vi "apolin.vi"() -> ()   [LabVIEW 2014]
uses:
  <vilib>/Platform/TimedLoop/XDataNode/timing_clust.ctl
  <vilib>/Platform/TimedLoop/XDataNode/nitl_modes.ctl
  <vilib>/Platform/TimedLoop/XDataNode/wakeup.ctl
  <vilib>/myRIO/Instrument Drivers/Onboard IO/AO/typedefs/AO Reference.ctl
  <vilib>/myRIO/Common/Instrument Driver Framework/Utilities/typedefs/myRIO Generic Hardware Reference.ctl
  <vilib>/myRIO/Common/Instrument Driver Framework/Utilities/typedefs/Hardware Version Enum.ctl
  <vilib>/myRIO/Common/Instrument Driver Framework/Utilities/typedefs/myRIO v1.0 Reference.ctl
  <vilib>/myRIO/Common/Instrument Driver Framework/Utilities/typedefs/Generic FPGA Reference.ctl
  <vilib>/myRIO/Common/Instrument Driver Framework/myRIO v1.0/AO/typedefs/AO Channels List.ctl
  <vilib>/myRIO/Common/Instrument Driver Framework/myRIO v1.0/AO/typedefs/AO Channels Enum.ctl
  <vilib>/myRIO/Common/Instrument Driver Framework/Utilities/typedefs/Analog Scaling Constants List.ctl
  <vilib>/myRIO/Common/Instrument Driver Framework/Utilities/typedefs/Analog Scaling Constants.ctl
  <vilib>/userdefined/High Color/nirio_resource_hc.ctl
  <vilib>/myRIO/Common/Instrument Driver Framework/myRIO v1.0/AO/vis/myRIO v1.1 Open AO.vi
  <vilib>/myRIO/Common/Instrument Driver Framework/Utilities/vis/Validate Channels.vi
  <vilib>/myRIO/Common/Instrument Driver Framework/myRIO v1.0/AO/vis/myRIO v1.0 Reserve AO.vi
  <vilib>/myRIO/Common/Instrument Driver Framework/myRIO v1.0/AO/vis/myRIO v1.0 Close AO.vi
  <vilib>/myRIO/Common/Instrument Driver Framework/myRIO v1.0/AO/vis/myRIO v1.0 Build MUX Configuration AO.vi
  <vilib>/myRIO/Common/Instrument Driver Framework/myRIO v1.0/Resource Manager/vis/myRIO v1.0 Reserve Channel List.vi
  <vilib>/myRIO/Common/Instrument Driver Framework/myRIO v1.0/AO/vis/myRIO v1.0 Unreserve AO.vi
  <vilib>/myRIO/Common/Instrument Driver Framework/myRIO v1.0/Resource Manager/vis/myRIO v1.0 Reserve Channel.vi
  <vilib>/myRIO/Common/Instrument Driver Framework/myRIO v1.0/Resource Manager/vis/myRIO v1.0 Unreserve Channel.vi
  <vilib>/myRIO/Common/Instrument Driver Framework/myRIO v1.0/Resource Manager/vis/myRIO v1.0 Unreserve Channel List.vi
  <vilib>/myRIO/Common/Instrument Driver Framework/myRIO v1.0/Resource Manager/vis/myRIO v1.0 Build Mutex Name.vi
  <vilib>/Utility/VariantDataType/GetNumericInfo.vi
  <vilib>/Utility/error.llb/Error Cluster From Error Code.vi
  <vilib>/myRIO/Common/Instrument Driver Framework/myRIO v1.0/myRIO v1.1 Open.vi
  <vilib>/myRIO/Common/Instrument Driver Framework/myRIO v1.0/AO/vis/myRIO v1.0 Get Scaling Constants AO.vi
  <vilib>/myRIO/Common/Instrument Driver Framework/Utilities/vis/IO Manager.vi
  <vilib>/myRIO/Common/Instrument Driver Framework/Utilities/vis/Configuration Manager.vi
  <vilib>/myRIO/Common/Instrument Driver Framework/myRIO v1.0/myRIO v1.0 Close.vi
  <vilib>/myRIO/Common/Instrument Driver Framework/myRIO v1.0/AO/vis/myRIO v1.0 Write AO.vi
  <vilib>/myRIO/Instrument Drivers/Onboard IO/AO/vis/myRIO AO Open.xnode
  <vilib>/platform/TimedLoop/XDataNode/XDataNode.xnode
  <vilib>/myRIO/Common/Instrument Driver Framework/myRIO v1.0/AI/typedefs/AI Channels Enum.ctl
  <vilib>/myRIO/Common/Instrument Driver Framework/myRIO v1.0/AI/typedefs/AI Channels List.ctl
  <vilib>/myRIO/Instrument Drivers/Onboard IO/AI/typedefs/AI Reference.ctl
  <vilib>/myRIO/Instrument Drivers/Onboard IO/AI/AI.lvlib
  <vilib>/myRIO/Common/Instrument Driver Framework/myRIO v1.0/AI/vis/myRIO v1.1 Open AI.vi
  <vilib>/myRIO/Instrument Drivers/Onboard IO/AI/vis/myRIO AI Open.xnode
  <vilib>/Platform/TimedLoop/XDataNode/XDNodeRunTimeDep.lvlib
  <vilib>/myRIO/Instrument Drivers/Onboard IO/AO/AO.lvlib
  <vilib>/measure/NI_MABase.lvlib
panel:
  out "x/y":dbl
  in  "Start \nPlayback":bool
  out "Recording 3":dbl[](graph)
  out "Array 3":dbl[][](array[numeric])
  in  "sampling info":cluster{"Fs":dbl, "#s":dbl}={"Fs"=40000.0, "#s"=40000.0} {"Fs" format="%.2p"}
  out "error out":errorcluster
  out "dt":dbl
  in  "tones":T1(array[cluster])=[{"frequency"=10.0, "amplitude"=1.0, "phase"=0.0}, {"frequency"=20.0, "amplitude"=0.1, "phase"=0.0}] {"phase" format="%.2p"; "amplitude" format="%0.2p"; "frequency" format="%0.2p"}
  in  "Stop \nPlaying":bool
  out "Array":dbl[](array[numeric])
  out "Recording 2":dbl(graph)
  in  "Stop \nRecording 2":bool
  out "Array 2":dbl[](array[numeric])
  in  "Start\nRecording 2":bool
  out "Recording 1":dbl[](graph)
  in  "Start/Stop\nRecording 1":bool
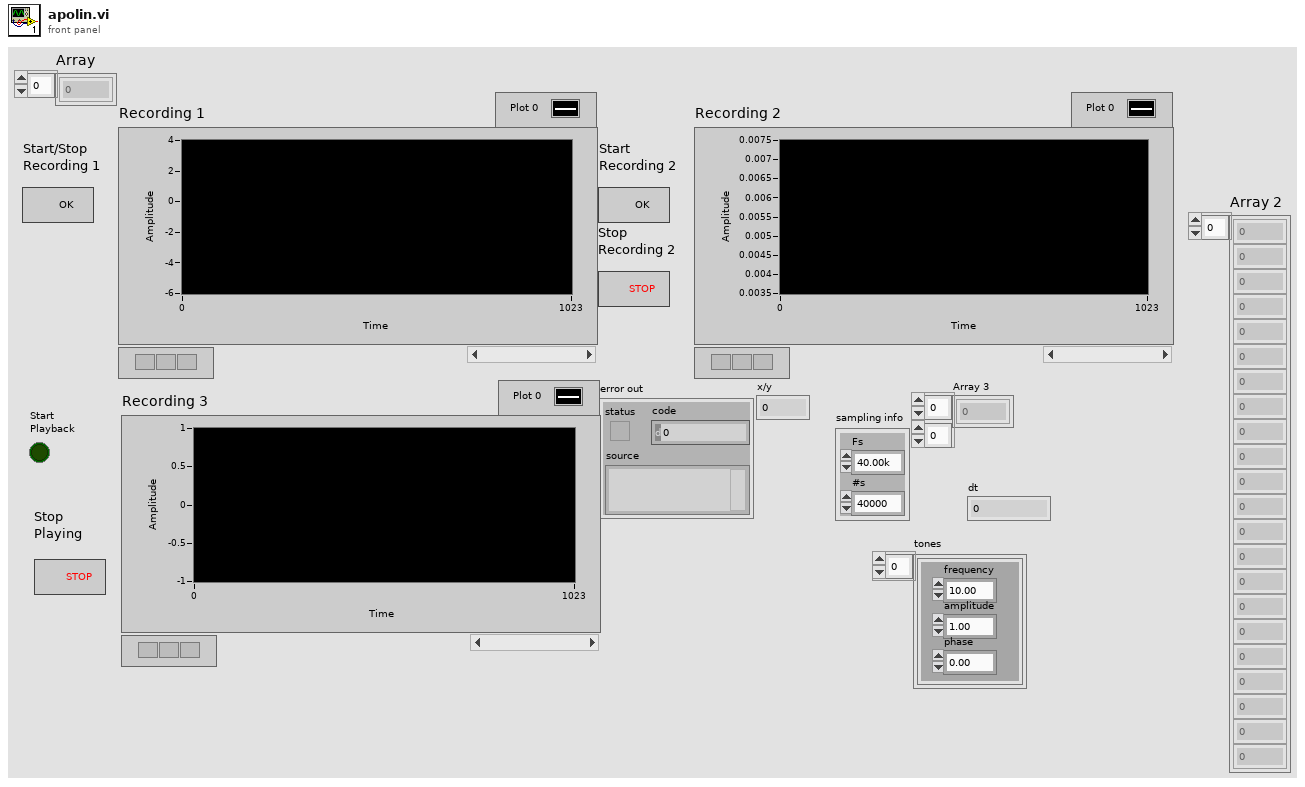
[diagram p1: front panel]
types:
  T1 = cluster{"frequency":dbl, "amplitude":dbl, "phase":dbl}[]
  T2 = typedef "XDNodeRunTimeDep.lvlib/timing_clust.ctl" = cluster{"Expected End [f-1]":u64, "Actual End [f-1]":u64, "Finished Late? [f-1]":bool, "Expected End [i-1]":u64, "Actual End [i-1]":u64, "Finished Late? [i-1]":bool, "Expected Start [i]":u64, "Actual Start [i]":u64, "Expected Start [f]":u64, "Actual Start [f]":u64, "Source Name":string, "Structure Name":string, "Period":i64, "Deadline":i64, "Offset":i64, "Start":i64, "Priority":i32, "Timeout":i32, "Mode":T3, "Wakeup Reason":T4, "Error":errorcluster, "Source Type":string, "Secondary Source Type":string, "Global End Time":u64, "Global Start Time":u64, "Frame Duration":u64, "Iteration Duration":u64, "Assigned CPU":i32, "I/O Scan Engine Mode":u32}
  T3 = typedef "XDNodeRunTimeDep.lvlib/nitl_modes.ctl" = enum32{"No Change", "Process missed periods, maintain original phase", "Discard missed periods, maintain original phase", "Process missed periods, ignore original phase", "Discard missed periods, ignore original phase"}
  T4 = typedef "XDNodeRunTimeDep.lvlib/wakeup.ctl" = enum32{"Normal", "Aborted", "Asynchronous wakeup", "Timing source error", "Timed loop error", "Timeout"}
  T5 = typedef "nirio_resource_hc.ctl" = tag
  T6 = typedef "Hardware Version Enum.ctl" = enum16{"Unknown", "myRIO-1900", "myRIO-1950"}
  T7 = typedef "AI.lvlib/AI Reference.ctl" = cluster{"myRIO Reference":T8, "AI Channels List":T11, "AI Scaling Constants List":T13}
  T8 = typedef "myRIO Generic Hardware Reference.ctl" = cluster{"myRIO Model":T6, "myRIO Hardware Reference":T9}
  T9 = typedef "myRIO v1.0 Reference.ctl" = cluster{"Generic FPGA Reference":T10, "Allow multiple opens":bool}
  T10 = typedef "Generic FPGA Reference.ctl" = refnum<k20>
  T11 = typedef "AI Channels List.ctl" = T12[]
  T12 = typedef "AI Channels Enum.ctl" = enum16{"Not Connected", "AudioIn/Left", "AudioIn/Right", "C/AI0", "C/AI1", "A/AI0", "A/AI1", "A/AI2", "A/AI3", "B/AI0", "B/AI1", "B/AI2", "B/AI3"}
  T13 = typedef "Analog Scaling Constants List.ctl" = T14[]
  T14 = typedef "Analog Scaling Constants.ctl" = cluster{"LSB Weight (Volts)":dbl, "Offset (Volts)":dbl, "Signed?":bool}
  T15 = typedef "AO.lvlib/AO Reference.ctl" = cluster{"myRIO Reference":T8, "AO Channel List":T16, "AO Scaling Constant List":T13}
  T16 = typedef "AO Channels List.ctl" = T17[]
  T17 = typedef "AO Channels Enum.ctl" = enum16{"Not Connected", "AudioOut/Left", "AudioOut/Right", "C/AO0", "C/AO1", "A/AO0", "A/AO1", "B/AO0", "B/AO1"}
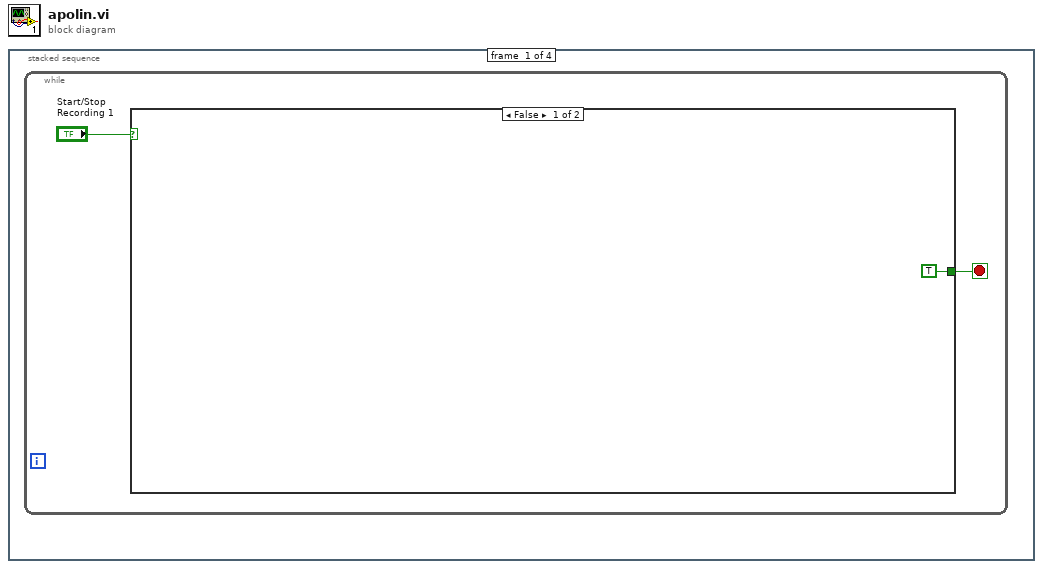
[diagram p0: block diagram]
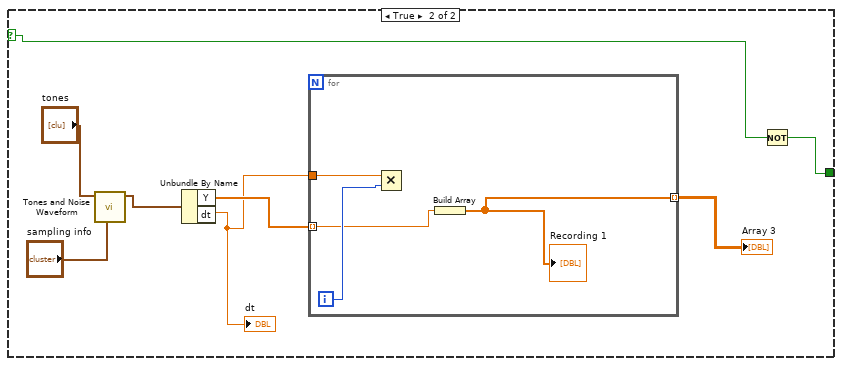
[diagram p2: hidden frame]
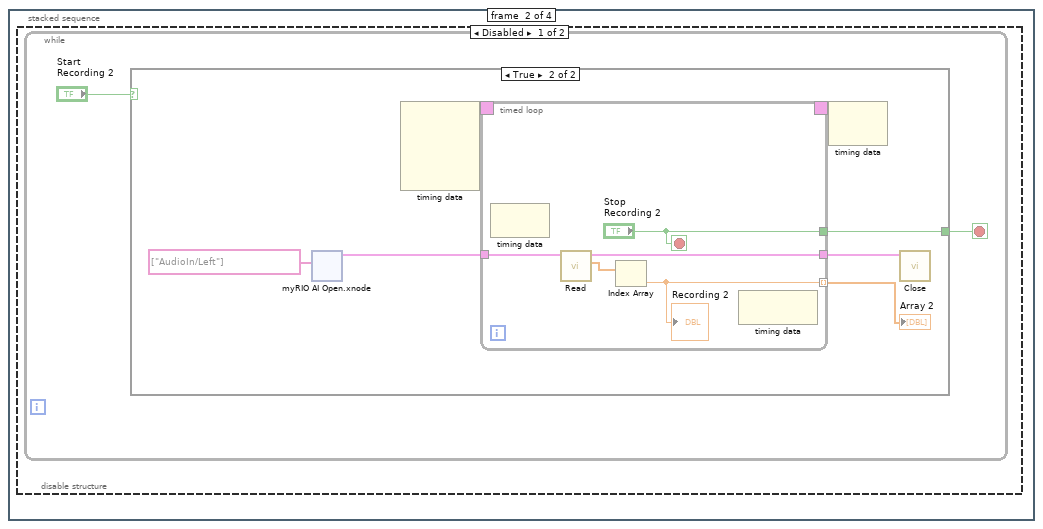
[diagram p3: hidden frame]
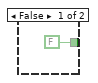
[diagram p4: hidden frame]
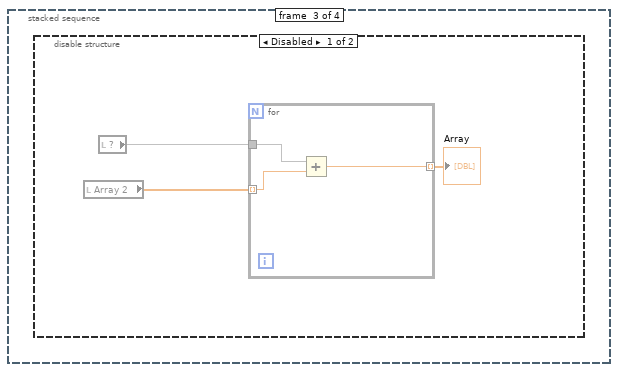
[diagram p6: hidden frame]
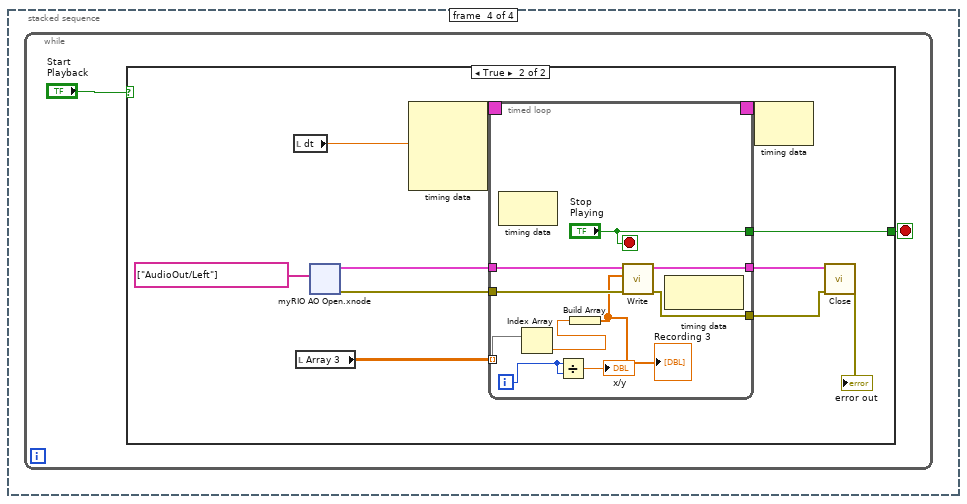
[diagram p8: hidden frame]
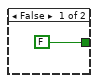
[diagram p9: hidden frame]
diagram:
  n1 = stacked-sequence {
    frame #0 {
      n2 = while {
        stop <- w2 stop-if-true
        n3 = case shown="False" "Start/Stop\nRecording 1" {
          selector: "Start/Stop\nRecording 1" -> [_ w4]
          tunnel: [TRUE ("stop recording") w5] -> w2
          frame False {
          }
          frame True {
            n4 = call <vilib>:"Tones and Noise Waveform.vi"("sampling info"="sampling info", "tones"="tones") -> ("signal out"=w10:waveform(dbl))  [unwired: 8 in, 1 out]
            n5 = Unbundle By Name(w10) -> ("Y"=w8:dbl[], "dt"=w7:dbl)
            "dt" <- w7
            n6 = for {
              tunnel: w8 -> [w13] mode=indexing
              tunnel: w7 -> [w15]
              tunnel: [w12] -> w6 mode=indexing
              i -> [w14]
              n7 = Multiply(x=w15, y=w14) -> ()  [unwired: 1 out]
              n8 = Build Array(w13) -> (w12:dbl[])
              "Recording 1" <- w12
            }
            "Array 3" <- w6
            n9 = Not(x=w4) -> (.not. x?=w5:bool)
          }
        }
      }
    }
    frame #1 {
      n10 = disable-structure shown="Disabled" {
        frame Disabled {
          n11 = while {
            stop <- w17 stop-if-true
            n12 = case shown="True" "Start\nRecording 2" {
              tunnel: [FALSE ("stop recording") w21] -> w17
              frame False {
              }
              frame True {
                n13 = xnode "myRIO AI Open.xnode"("Channel Names"=tag[] ["AudioIn/Left"]) -> ("AI Ref Out"=w22:T7)  [unwired: 2 in, 1 out]
                n14 = node-c288() -> (w25:T2)  [unwired: 4 in]
                n15 = timed-loop {
                  timing: w25 -> [_]
                  timing-out: [_] -> w24
                  tunnel: [w27] -> w19 mode=indexing
                  tunnel: ["Stop \nRecording 2"] -> w21
                  tunnel: w22 -> [w30]
                  tunnel: [w29] -> w20
                  stop <- "Stop \nRecording 2" stop-if-true
                  n16 = node-c288() -> ()  [unwired: 1 in, 1 out]
                  n17 = call <vilib>:"Read.vi"("AI Ref In"=w30) -> ("Values"=w28:dbl[], "AI Ref Out"=w29:T7)  [unwired: 8 in, 1 out]
                  n18 = Index Array(array=w28) -> (element=w27:dbl)  [unwired: 1 in]
                  "Recording 2" <- w27
                  n19 = node-c288() -> ()  [unwired: 1 in, 1 out]
                }
                "Array 2" <- w19
                n20 = node-c288(w24) -> ()  [unwired: 1 out]
                n21 = call <vilib>:"Close.vi"("AI Ref In"=w20) -> ()  [unwired: 10 in, 1 out]
              }
            }
          }
        }
        frame Enabled {
        }
      }
    }
    frame #2 {
      n22 = disable-structure shown="Disabled" {
        frame Disabled {
          n23 = local read "Array 2"() -> (w54:dbl[])
          n24 = local read item#-1() -> (w55)
          n25 = for {
            tunnel: w55 -> [w57]
            tunnel: w54 -> [w58] mode=indexing
            tunnel: [w56] -> w53 mode=indexing
            n26 = Add(x=w57, y=w58) -> (x+y=w56:dbl)
          }
          "Array" <- w53
        }
        frame Enabled {
        }
      }
    }
    frame #3 {
      n27 = while {
        stop <- w60 stop-if-true
        n28 = case shown="True" "Start \nPlayback" {
          tunnel: [FALSE ("stop playing") w66] -> w60
          frame False {
          }
          frame True {
            n29 = local read "dt"() -> (w62:dbl)
            n30 = local read "Array 3"() -> (w67:dbl[][])
            n31 = xnode "myRIO AO Open.xnode"("Channel Names"=tag[] ["AudioOut/Left"]) -> ("error out"=w65:errorcluster, "AO Ref Out"=w70:T15)  [unwired: 2 in]
            n32 = node-c288(w62) -> (w72:T2)  [unwired: 3 in]
            n33 = timed-loop {
              timing: w72 -> [_]
              timing-out: [_] -> w71
              tunnel: [w100] -> w69
              tunnel: w70 -> [w99]
              tunnel: w67 -> [w95] mode=indexing
              tunnel: ["Stop \nPlaying"] -> w66
              tunnel: w65 -> [w97]
              tunnel: [w96] -> w64
              i -> [w92]
              stop <- "Stop \nPlaying" stop-if-true
              n34 = node-c288() -> ()  [unwired: 1 in, 1 out]
              n35 = Index Array(array=w95) -> (element=w94:dbl)  [unwired: 1 in]
              n36 = Divide(x=w92, y=w92) -> (x/y=→"x/y":dbl)
              n37 = Build Array(w94) -> (w93:dbl[])
              "Recording 3" <- w93
              n38 = call <vilib>:"Write.vi"("error in (no error)"=w97, "Values"=w93, "AO Ref In"=w99) -> ("error out"=w96:errorcluster, "AO Ref Out"=w100:T15)  [unwired: 6 in]
              n39 = node-c288() -> ()  [unwired: 1 in, 1 out]
            }
            n40 = node-c288(w71) -> ()  [unwired: 1 out]
            n41 = call <vilib>:"Close.vi"("error in (no error)"=w64, "AO Ref In"=w69) -> ("error out"=→"error out":errorcluster)  [unwired: 9 in]
          }
        }
      }
    }
  }
